vi "Faill_adding_value.vi"(9 "index":i32=31, 10 "input array":string[](array[string]), 11 "Boolean":bool) -> (3 "output array":string[](array[string]))   [LabVIEW 2021]
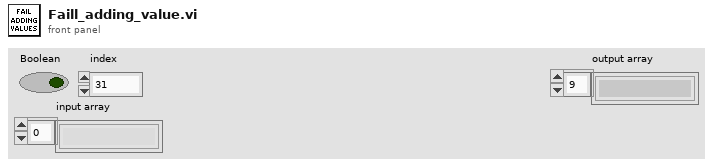
[diagram p1: front panel]
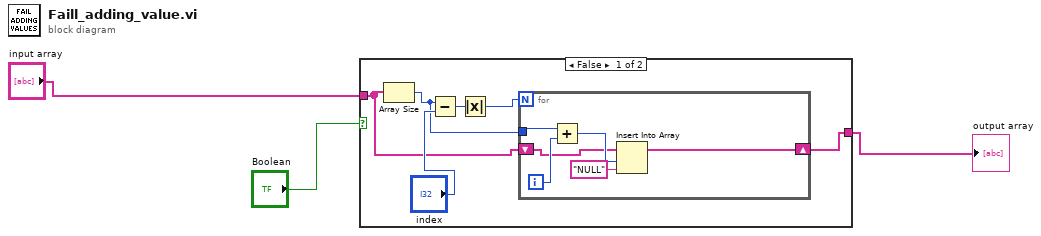
[diagram p0: block diagram]
diagram:
  n1 = case shown="False" "Boolean" {
    tunnel: [w6 w16] -> w2
    tunnel: "input array" -> [w4 w16]
    frame False {
      n2 = Array Size(array=w4) -> (size(s)=w7:i32)
      n3 = Subtract(x=w7, y="index") -> (x-y=w8:i32)
      n4 = Absolute Value(x=w8) -> (abs(x)=w5:i32)
      n5 = for {
        N: w5 -> [_]
        tunnel: w7 -> [w15]
        shift-right: [w11] -> w6
        shift-left: w4 -> [w10]
        i -> [w14]
        n6 = Add(x=w15, y=w14) -> (x+y=w13:i32)
        n7 = Insert Into Array(array=w10, index=w13, new element="NULL" ("new element/subarray")) -> (w11:string[])
      }
    }
    frame True {
    }
  }
  "output array" <- w2
